vi "StringSubset.vi"() -> ()   [LabVIEW 2019]
panel:
  out "Str2":string
  out "Str1":string
  in  "String1":string="Pomogranate"
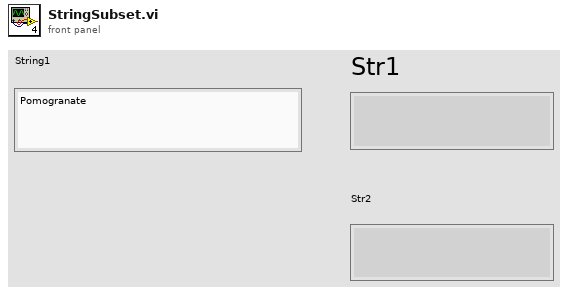
[diagram p1: front panel]
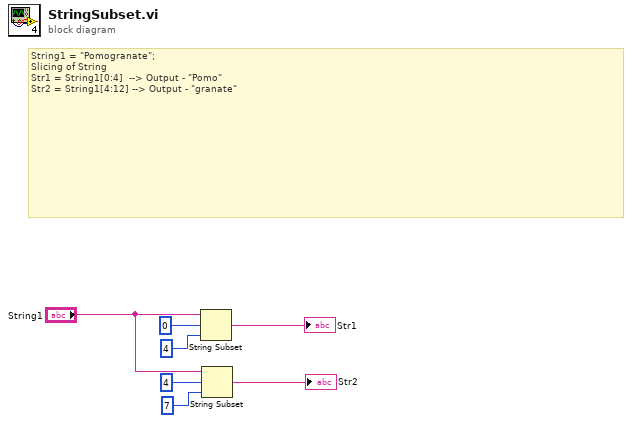
[diagram p0: block diagram]
diagram:
  # "String1 = \"Pomogranate\";\nSlicing of String\nStr1 = String1[0:4]  --> Output - \"Pomo\"\nStr2 = String1[4:12] --> Output - \"granate\""
  n1 = String Subset(string="String1", offset (0)=0, length (rest)=4 ("length (rest)")) -> (substring=→"Str1":string)
  n2 = String Subset(string="String1", offset (0)=4, length (rest)=7 ("length (rest)")) -> (substring=→"Str2":string)
